vi "DataTranslation_old.vi"() -> (15 "error out":errorcluster={"status"=TRUE, "code"=1172, "source"="Error calling method LvLink2.LvTask.ReadDblData2DAs1D, (System.Reflection.TargetInvocationException: Exception has been thrown by the target of an invocation.\n\tInner Exception: LvLink2.LvException: Timeout) <append><b>LvLink2.LvException</b> in OLReadMultiple2D.vi->DataTranslation_server.vi->Acquire_Data.vi->Get_data.vi->Measurement.vi"})   [LabVIEW 2011]
uses:
  Data_Translation/DataTranslation_global.vi
  Globals/Meas_global.vi
  PWA/PWAtasksGLOBAL.vi
  <userlib>/LV-Link3/PolySubVIs/DtCreateAinChan.vi
  <userlib>/LV-Link3/PolySubVIs/DtOLTimingSetInput.vi
  <userlib>/LV-Link3/PolySubVIs/DtOLReadMultiple2D.vi
  <userlib>/LV-Link3/PolySubVIs/DtOLTriggerDigital.vi
panel:
  in  "error in":errorcluster
  out "AFG error out":errorcluster
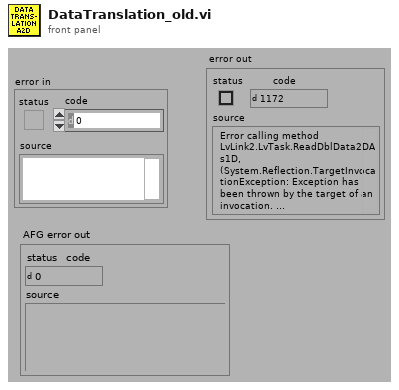
[diagram p1: front panel]
types:
  T1 = typedef "Ch_and_Spans.ctl" = cluster{"high limit (10V)":sgl, "low limit (-10V)":sgl, "Ch No":i16, "Var name":string, "Use Latest Calib":bool}
  T2 = typedef "Trigger_Mode.ctl" = enum16{"Free Running", "Start on Trigger", "Trigger Every Block", "Trigger Every Sample"}
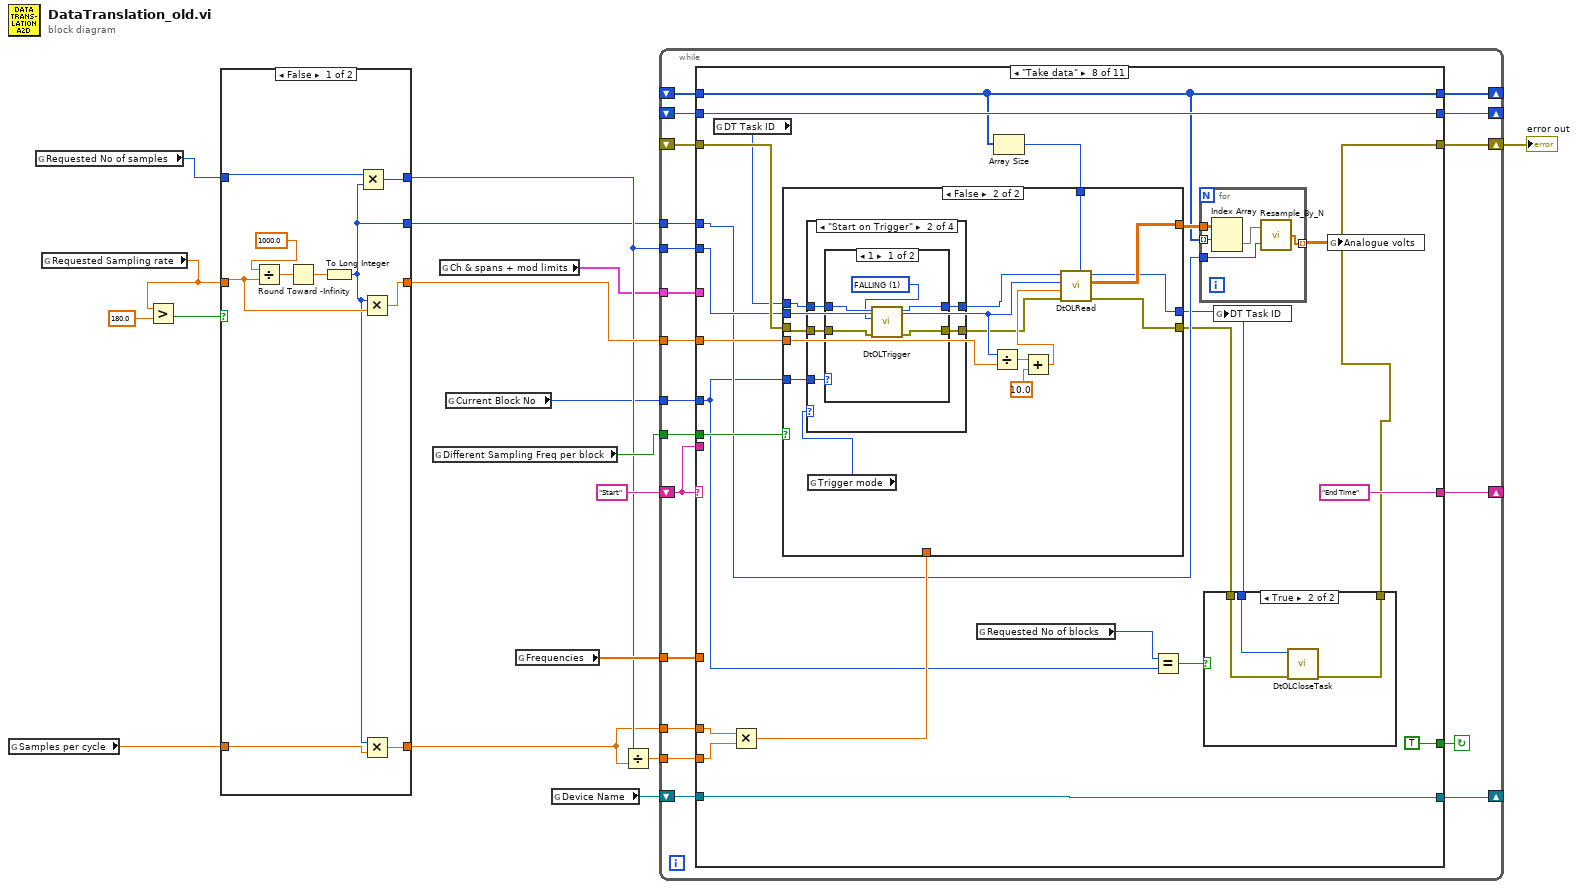
[diagram p0: block diagram]
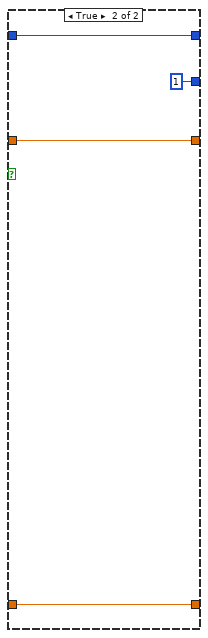
[diagram p2: hidden frame]
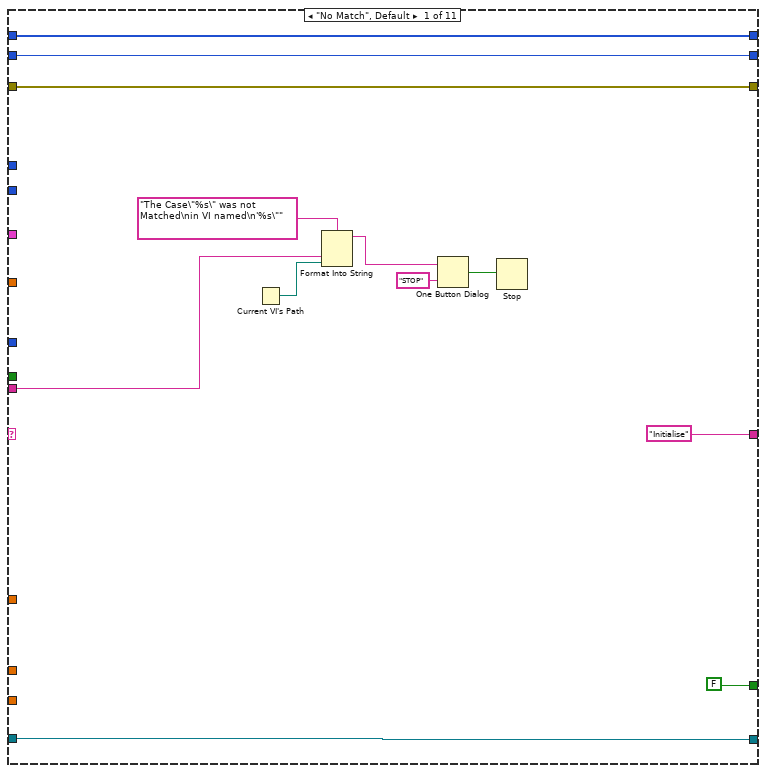
[diagram p3: hidden frame]
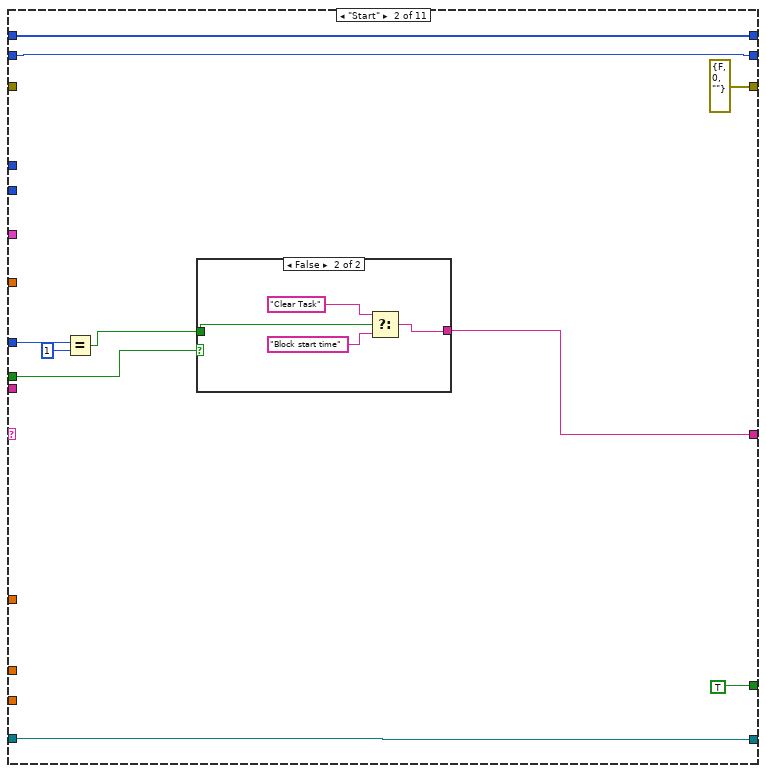
[diagram p4: hidden frame]
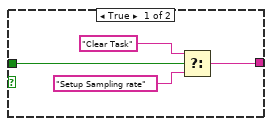
[diagram p5: hidden frame]
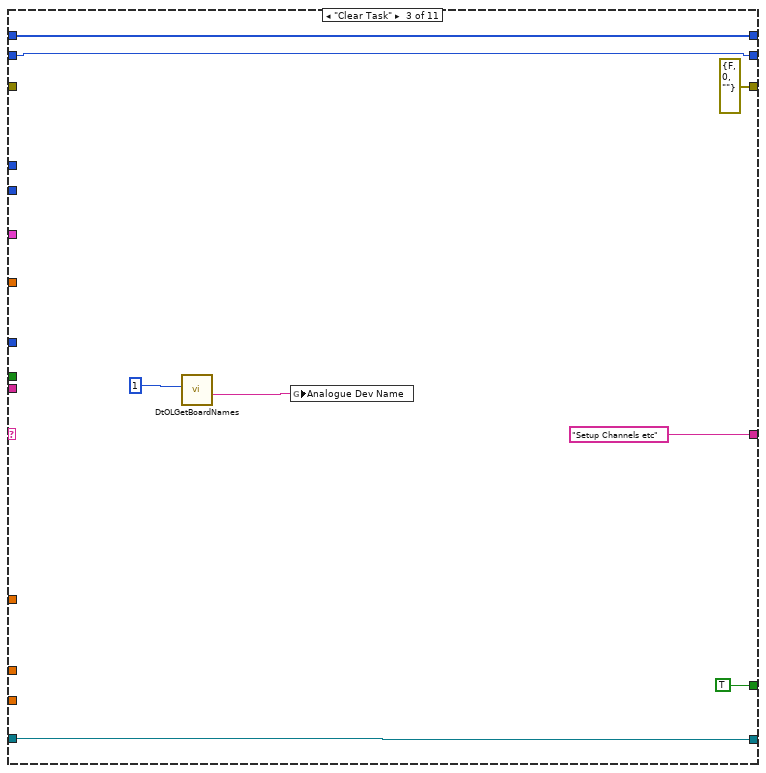
[diagram p6: hidden frame]
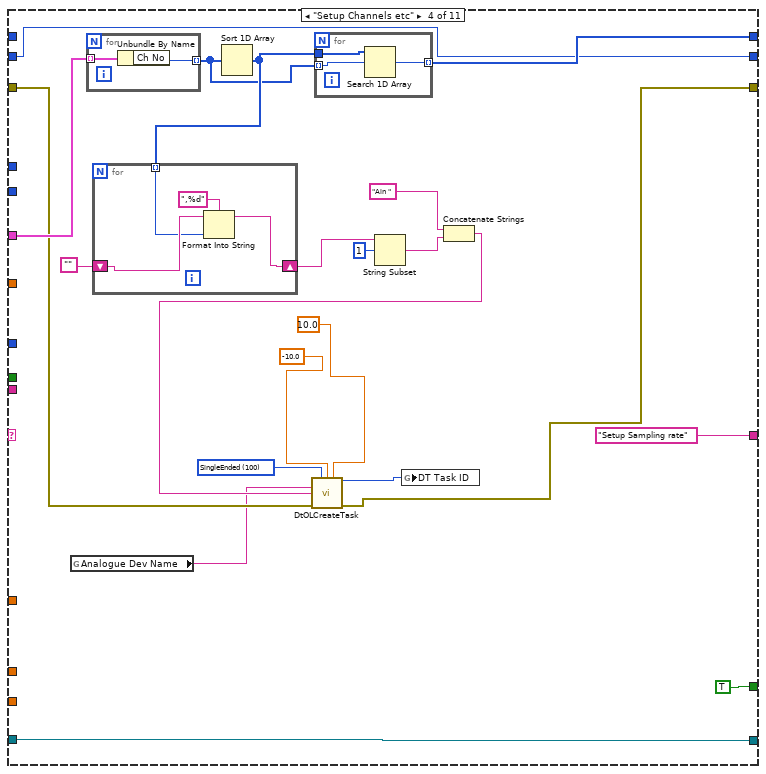
[diagram p7: hidden frame]
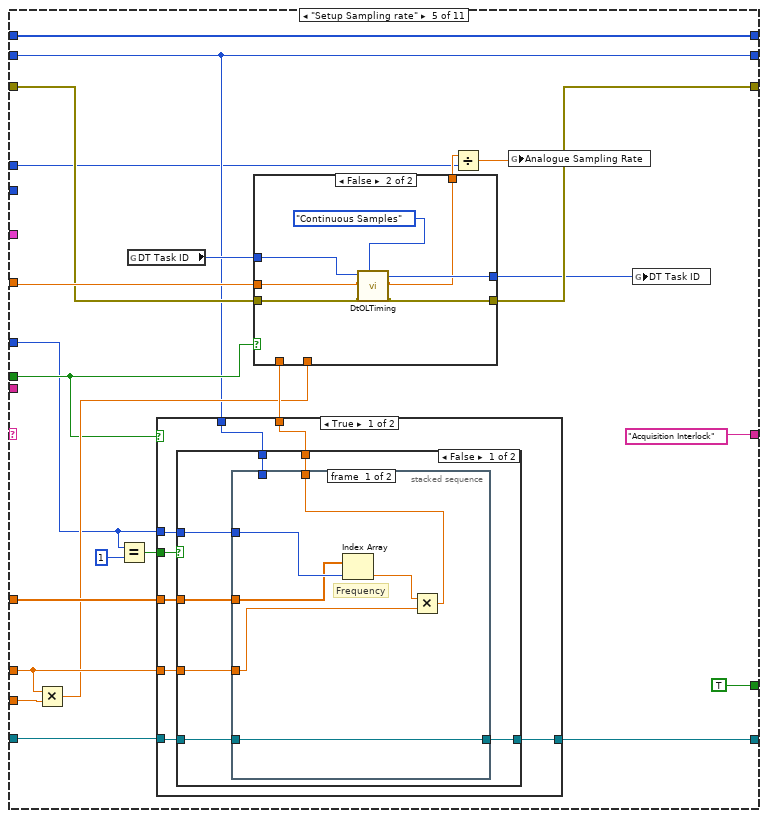
[diagram p8: hidden frame]
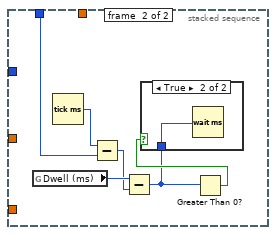
[diagram p9: hidden frame]
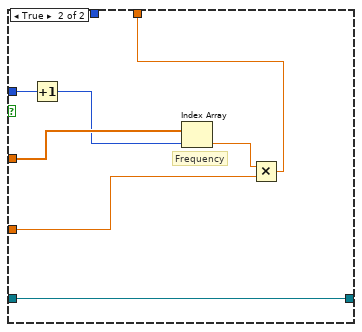
[diagram p11: hidden frame]
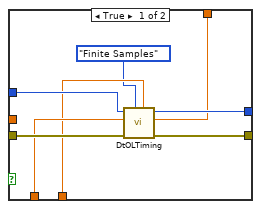
[diagram p13: hidden frame]
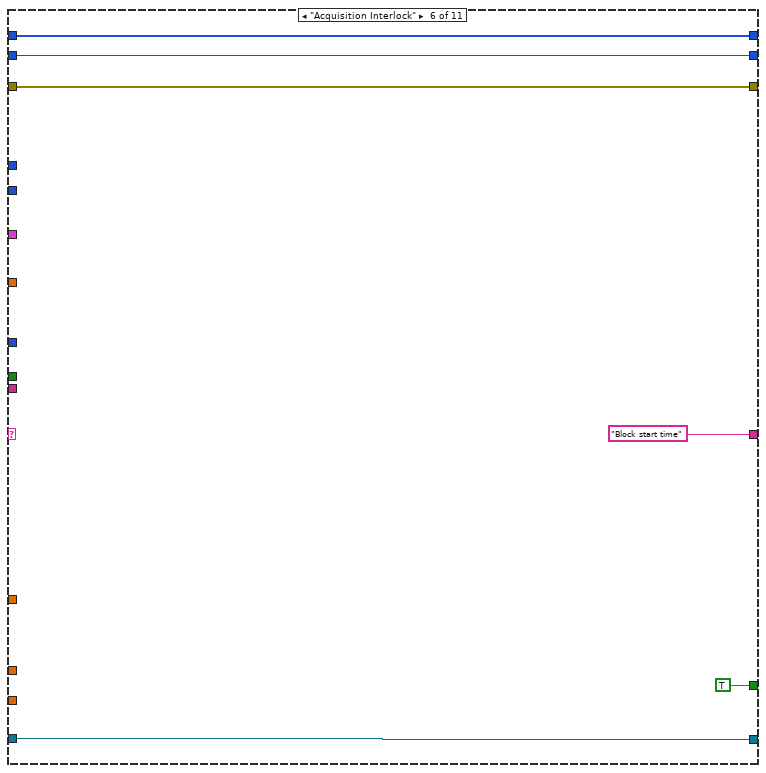
[diagram p14: hidden frame]
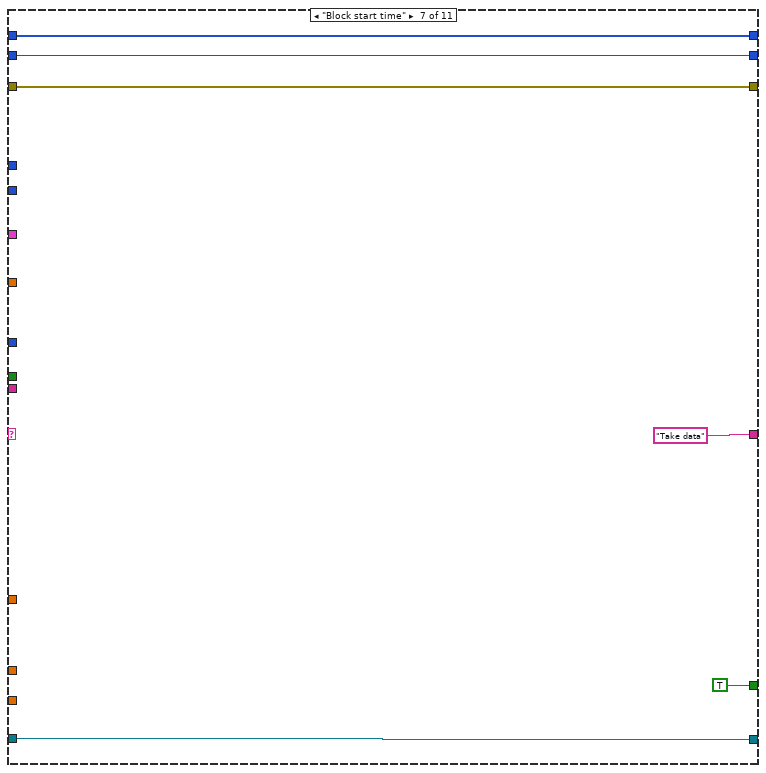
[diagram p15: hidden frame]
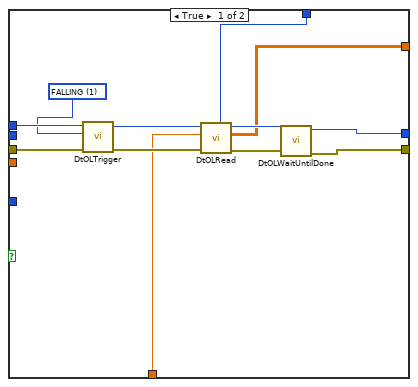
[diagram p17: hidden frame]
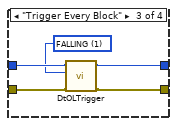
[diagram p20: hidden frame]
diagram:
  n1 = global read "DataTranslation_global.vi" "Samples per cycle"() -> (w6:dbl)
  n2 = global read "Meas_global.vi" "Requested No of samples"() -> (w2:i32)
  n3 = global read "Meas_global.vi" "Requested Sampling rate"() -> (w3:dbl)
  n4 = Greater?(x=w3, y=180.0) -> (0:w10:bool)
  n5 = case shown="False" w10 {
    tunnel: w3 -> [w21 w31]
    tunnel: [w22 w31] -> w9
    tunnel: [w24 w30] -> w8
    tunnel: w2 -> [w23 w30]
    tunnel: [w20 w29] -> w7
    tunnel: w6 -> [w19 w29]
    tunnel: [w18 1] -> w5
    frame False {
      n6 = Divide(x=1000.0, y=w21) -> (x/y=w26:dbl)
      n7 = Round Toward -Infinity(1:w26) -> (0:w25:dbl)
      n8 = To Long Integer(number=w25) -> (32bit integer=w18:i32)
      n9 = Multiply(x=w23, y=w18) -> (x*y=w24:i32)
      n10 = Multiply(x=w18, y=w21) -> (x*y=w22:dbl)
      n11 = Multiply(x=w18, y=w19) -> (x*y=w20:dbl)
    }
    frame True {
    }
  }
  n12 = global read "DataTranslation_global.vi" "Different Sampling Freq per block"() -> (w12:bool)
  n13 = global read "Meas_global.vi" "Ch & spans + mod limits"() -> (w4:T1[])
  n14 = global read "Meas_global.vi" "Current Block No"() -> (w1:i32)
  n15 = global read "DataTranslation_global.vi" "Frequencies"() -> (w13:dbl[])
  n16 = global read "DataTranslation_global.vi" "Device Name"() -> (w14:refnum<visa-resource-name>)
  n17 = Divide(x=w8, y=w7) -> (x/y=w15:dbl)
  n18 = while {
    shift-left: "Start" -> [w49]
    shift-right: [w50] -> _
    shift-right: [w43] -> w16
    shift-left: _ -> [w48]
    tunnel: w9 -> [w47]
    tunnel: w8 -> [w46]
    tunnel: w1 -> [w45]
    tunnel: w4 -> [w44]
    shift-right: [w42] -> _
    shift-left: _ -> [w41]
    tunnel: w7 -> [w39]
    shift-right: [w38] -> _
    shift-left: w14 -> [w40]
    tunnel: w15 -> [w37]
    tunnel: w12 -> [w36]
    tunnel: w13 -> [w35]
    shift-right: [w34] -> _
    shift-left: _ -> [w33]
    tunnel: w5 -> [w32]
    stop <- w51 continue-if-true
    n19 = case shown="\"Take data\"" w49 {
      tunnel: [FALSE TRUE TRUE TRUE TRUE TRUE TRUE TRUE w289 FALSE FALSE] -> w51
      tunnel: ["Initialise" w72 "Setup Channels etc" "Setup Sampling rate" "Acquisition Interlock" "Block start time" "Take data" "End Time" "Add info to block header" ("f") "End" ("f") "End" ("f")] -> w50
      tunnel: w49 -> [w58 _ _ _ _ _ _ _ _ _ _]
      tunnel: [w55 errorcluster {"status"=FALSE, "code"=0, "source"=""} ("error out") errorcluster {"status"=FALSE, "code"=0, "source"=""} ("error out") w92 w141 w199 w206 w209 w291 w304 w335] -> w43
      tunnel: w48 -> [w55 _ _ w93 w139 w199 w206 w227 w291 w304 w335]
      tunnel: w47 -> [_ _ _ _ w140 _ _ w223 _ _ _]
      tunnel: w46 -> [_ _ _ _ _ _ _ w224 _ _ _]
      tunnel: w45 -> [_ w66 _ _ w121 _ _ w207 _ w297 _]
      tunnel: w44 -> [_ _ _ w103 _ _ _ _ _ _ _]
      tunnel: [w54 w70 w87 w100 w136 w197 w203 w216 w290 w303 w334] -> w42
      tunnel: w41 -> [w54 w70 w87 _ w136 w197 w203 w216 w290 w303 w334]
      tunnel: w40 -> [w53 w69 w86 w99 w133 w196 w202 w222 w288 w302 w333]
      tunnel: w35 -> [_ _ _ _ w135 _ _ _ _ w300 _]
      tunnel: w39 -> [_ _ _ _ w129 _ _ w220 _ _ _]
      tunnel: [w53 w69 w86 w99 w132 w196 w202 w222 w288 w301 w333] -> w38
      tunnel: w37 -> [_ _ _ _ w130 _ _ w221 _ _ _]
      tunnel: w36 -> [_ w68 _ _ w127 _ _ w218 w289 _ _]
      tunnel: [w52 w67 w85 w98 w126 w195 w201 w217 w287 w298 w332] -> w34
      tunnel: w33 -> [w52 w67 w85 w98 w126 w195 w201 w217 w287 _ w332]
      tunnel: w32 -> [_ _ _ _ w123 _ _ w214 _ _ _]
      frame "No Match", Default {
        n20 = Current VI's Path() -> (path=w57:path)
        n21 = Format Into String(format string="The Case\"%s\" was not Matched\nin VI named\n'%s\"" ("Format String"), w58, w57) -> (resulting string=w61:string)  [unwired: 2 in, 1 out]
        n22 = One Button Dialog(message=w61, button name ("OK")="STOP") -> (true=w59:bool)
        n23 = Stop(stop? (T)=w59) -> ()
      }
      frame "Start" {
        n24 = Equal?(x=w66, y=1) -> (x = y?=w64:bool)
        n25 = case shown="False" w68 {
          tunnel: w64 -> [w75 w79]
          tunnel: [w74 w78] -> w72
          frame True {
            n26 = Select(t="Clear Task", s=w75, f="Setup Sampling rate") -> (s? t:f=w74:string)
          }
          frame False {
            n27 = Select(t="Clear Task", s=w79, f="Block start time") -> (s? t:f=w78:string)
          }
        }
      }
      frame "Clear Task" {
        n28 = call <userlib>:"DtOLGetBoardNames.vi"("Select Board"=u32 1) -> ("Board Name"=w83:string)  [unwired: 8 in, 2 out]
        n29 = global write "PWAtasksGLOBAL.vi" "Analogue Dev Name"(w83) -> ()
      }
      frame "Setup Channels etc" {
        w94 = 100 items=["SingleEnded"=100, "Differential"=101] ("Channel Type")
        n30 = global read "PWAtasksGLOBAL.vi" "Analogue Dev Name"() -> (w90:string)
        n31 = for {
          tunnel: w103 -> [w115] mode=indexing
          tunnel: [w114] -> w101 mode=indexing
          n32 = Unbundle By Name(w115) -> ("Ch No"=w114:i16)
        }
        n33 = Sort 1D Array(array=w101) -> (sorted array=w102:i16[])
        n34 = for {
          shift-right: [w117] -> w108
          shift-left: "" -> [w118]
          tunnel: w102 -> [w116] mode=indexing
          n35 = Format Into String(format string=",%d", initial string=w118, w116) -> (resulting string=w117:string)  [unwired: 1 in, 1 out]
        }
        n36 = for {
          tunnel: w102 -> [w113]
          tunnel: w101 -> [w112] mode=indexing
          tunnel: [w111] -> w100 mode=indexing
          n37 = Search 1D Array(1D array=w113, element=w112) -> (index of element=w111:i32)  [unwired: 1 in]
        }
        n38 = String Subset(string=w108, offset (0)=1) -> (substring=w105:string)  [unwired: 1 in]
        n39 = Concatenate Strings("Ain ", w105) -> (w97:string)
        n40 = call-poly <userlib>:"DtOLCreateTask.vi"("Channel Type"=w94, "Range Min"=-10.0, "Range Max"=10.0, "Board Name"=w90, "Channel"=w97, "error in (no error)"=w93) -> ("Task out"=w91:i32, "error out"=w92:errorcluster)  [unwired: 7 in, 1 out]
        n41 = global write "DataTranslation_global.vi" "DT Task ID"(w91) -> ()
      }
      frame "Setup Sampling rate" {
        n42 = Multiply(x=w129, y=w130) -> (x*y=w128:dbl)
        n43 = Equal?(x=w121, y=1) -> (x = y?=w125:bool)
        n44 = global read "DataTranslation_global.vi" "DT Task ID"() -> (w137:i32)
        n45 = case shown="True" w127 {
          tunnel: w135 -> [w146 _]
          tunnel: [w150 w178] -> w134
          tunnel: w129 -> [w149 w178]
          tunnel: w121 -> [w148 _]
          tunnel: w133 -> [w147 w179]
          tunnel: [w145 w179] -> w132
          tunnel: w126 -> [w144 _]
          tunnel: w125 -> [w143 _]
          frame True {
            n46 = case shown="False" w143 {
              tunnel: [w157 w174] -> w150
              tunnel: w149 -> [w156 w173]
              tunnel: w148 -> [w151 w175]
              tunnel: w147 -> [w155 w172]
              tunnel: w146 -> [w154 w176]
              tunnel: [w153 w172] -> w145
              tunnel: w144 -> [w152 _]
              frame False {
                n47 = stacked-sequence {
                  tunnel: [w163 _] -> w157
                  tunnel: w156 -> [w162 _]
                  tunnel: w151 -> [w161 _]
                  tunnel: w155 -> [w158 _]
                  tunnel: w154 -> [w160 _]
                  tunnel: [w158 _] -> w153
                  tunnel: w152 -> [_ w168]
                  frame #0 {
                    # "Frequency"
                    n48 = Index Array(array=w160, index=w161) -> (element=w159:dbl)
                    n49 = Multiply(x=w159, y=w162) -> (x*y=w163:dbl)
                  }
                  frame #1 {
                    n50 = global read "DataTranslation_global.vi" "Dwell (ms)"() -> (w167:u32)
                    n51 = Tick Count (ms)() -> (millisecond timer value=w169:u32)
                    n52 = Subtract(x=w169, y=w168) -> (x-y=w166:u32)
                    n53 = Subtract(x=w167, y=w166) -> (x-y=w164:u32)
                    n54 = Greater Than 0?(x=w164) -> (x > 0?=w165:bool)
                    n55 = case shown="True" w165 {
                      tunnel: w164 -> [_ w170]
                      frame False {
                      }
                      frame True {
                        n56 = Wait (ms)(milliseconds to wait=w170) -> ()  [unwired: 1 out]
                      }
                    }
                  }
                }
              }
              frame True {
                # "Frequency"
                n57 = Increment(x=w175) -> (x+1=w171:i32)
                n58 = Index Array(array=w176, index=w171) -> (element=w177:dbl)
                n59 = Multiply(x=w177, y=w173) -> (x*y=w174:dbl)
              }
            }
          }
          frame False {
          }
        }
        n60 = case shown="False" w127 {
          tunnel: [w184 w189] -> w141
          tunnel: w140 -> [_ w192]
          tunnel: [w183 w191] -> w124
          tunnel: w139 -> [w185 w190]
          tunnel: [w186 w194] -> w138
          tunnel: w137 -> [w187 w193]
          tunnel: w134 -> [w182 _]
          tunnel: w128 -> [w181 _]
          frame True {
            n61 = call-poly <userlib>:"DtOLTiming.vi"("Samples Per Channel"=w181, "Sample Mode"=enum16{"Finite Samples", "Continuous Samples"}."Finite Samples", "error in (no error)"=w185, "Sample Freq (Hz)"=w182, "Task in"=w187) -> ("error out"=w184:errorcluster, "Actual Sample Freq"=w183:dbl, "Task out"=w186:i32)  [unwired: 3 in, 1 out]
          }
          frame False {
            n62 = call-poly <userlib>:"DtOLTiming.vi"("Sample Mode"=enum16{"Finite Samples", "Continuous Samples"}."Continuous Samples", "error in (no error)"=w190, "Sample Freq (Hz)"=w192, "Task in"=w193) -> ("error out"=w189:errorcluster, "Actual Sample Freq"=w191:dbl, "Task out"=w194:i32)  [unwired: 4 in, 1 out]
          }
        }
        n63 = Divide(x=w124, y=w123) -> (x/y=w122:dbl)
        n64 = global write "Meas_global.vi" "Analogue Sampling Rate"(w122) -> ()
        n65 = global write "DataTranslation_global.vi" "DT Task ID"(w138) -> ()
      }
      frame "Acquisition Interlock" {
      }
      frame "Block start time" {
      }
      frame "Take data" {
        n66 = global read "DataTranslation_global.vi" "DT Task ID"() -> (w226:i32)
        n67 = Multiply(x=w220, y=w221) -> (x*y=w219:dbl)
        n68 = global read "Meas_global.vi" "Requested No of blocks"() -> (w213:i32)
        n69 = Array Size(array=w216) -> (size(s)=w215:i32)
        n70 = case shown="False" w218 {
          tunnel: w227 -> [w245 w255]
          tunnel: [w242 w249] -> w210
          tunnel: [w239 w247] -> w212
          tunnel: w226 -> [w238 w256]
          tunnel: [w236 w248] -> w225
          tunnel: w224 -> [_ w252]
          tunnel: w223 -> [_ w260]
          tunnel: w219 -> [w235 _]
          tunnel: w207 -> [_ w254]
          tunnel: w215 -> [w234 w246]
          frame True {
            w237 = 1 items=["RISING", "FALLING"] ("External Trigger Polarity")
            n71 = call-poly <userlib>:"DtOLTrigger.vi"("error in (no error)"=w245, "External Trigger Polarity"=w237, "Task in"=w238) -> ("error out"=w244:errorcluster, "Task out"=w241:i32)  [unwired: 7 in]
            n72 = call-poly <userlib>:"DtOLRead.vi"("Number Chan to Read"=w234, "error in (no error)"=w244, "Samples Per Channel"=w235, "Task in"=w241) -> ("error out"=w243:errorcluster, "2D Data out"=w236:dbl[][], "Task out"=w240:i32)  [unwired: 3 in, 2 out]
            n73 = call <userlib>:"DtOLWaitUntilDone.vi"("error in"=w243, "Task in"=w240) -> ("error out"=w242:errorcluster, "Task out"=w239:i32)  [unwired: 8 in]
          }
          frame False {
            n74 = global read "Meas_global.vi" "Trigger mode"() -> (w257:T2)
            n75 = case shown="\"Start on Trigger\"" w257 {
              tunnel: [w262 w264 w278 w281] -> w253
              tunnel: w256 -> [w262 w266 w279 w281]
              tunnel: [w261 w263 w275 w280] -> w250
              tunnel: w255 -> [w261 w265 w276 w280]
              tunnel: w254 -> [_ w267 _ _]
              frame "Free Running" {
              }
              frame "Start on Trigger" {
                n76 = case shown="1" w267 {
                  tunnel: w266 -> [w272 w274]
                  tunnel: w265 -> [w270 w273]
                  tunnel: [w268 w274] -> w264
                  tunnel: [w269 w273] -> w263
                  frame 1 {
                    w271 = 1 items=["RISING", "FALLING"] ("External Trigger Polarity")
                    n77 = call-poly <userlib>:"DtOLTrigger.vi"("error in (no error)"=w270, "External Trigger Polarity"=w271, "Task in"=w272) -> ("error out"=w269:errorcluster, "Task out"=w268:i32)  [unwired: 7 in]
                  }
                  frame 2, Default {
                  }
                }
              }
              frame "Trigger Every Block" {
                w277 = 1 items=["RISING", "FALLING"] ("External Trigger Polarity")
                n78 = call-poly <userlib>:"DtOLTrigger.vi"("error in (no error)"=w276, "External Trigger Polarity"=w277, "Task in"=w279) -> ("error out"=w275:errorcluster, "Task out"=w278:i32)  [unwired: 7 in]
              }
              frame "Trigger Every Sample" {
              }
            }
            n79 = Divide(x=w252, y=w260) -> (x/y=w258:dbl)
            n80 = Add(x=w258, y=10.0) -> (x+y=w251:dbl)
            n81 = call-poly <userlib>:"DtOLRead.vi"("Number Chan to Read"=w246, "error in (no error)"=w250, "Timeout"=w251, "Samples Per Channel"=w252, "Task in"=w253) -> ("error out"=w249:errorcluster, "2D Data out"=w248:dbl[][], "Task out"=w247:i32)  [unwired: 2 in, 2 out]
          }
        }
        n82 = Equal?(x=w213, y=w207) -> (x = y?=w211:bool)
        n83 = for {
          tunnel: w216 -> [w286] mode=indexing
          tunnel: w225 -> [w285]
          tunnel: [w283] -> w208 mode=indexing
          tunnel: w214 -> [w282]
          n84 = Index Array(array=w285, index (row)=w286) -> (element=w284:dbl[])  [unwired: 1 in]
          n85 = call "Resample_By_N.vi"("Resample Factor"=w282, "Array In"=w284) -> ("Array Out"=w283:dbl[])
        }
        n86 = case shown="True" w211 {
          tunnel: w212 -> [_ w233]
          tunnel: w210 -> [w230 w232]
          tunnel: [w230 w231] -> w209
          frame False {
          }
          frame True {
            n87 = call <userlib>:"DtOLCloseTask.vi"("Error in"=w232, "Task in"=w233) -> ("Error Out"=w231:errorcluster)  [unwired: 9 in]
          }
        }
        n88 = global write "DataTranslation_global.vi" "DT Task ID"(w212) -> ()
        n89 = global write "Meas_global.vi" "Analogue volts"(w208) -> ()
      }
      frame "End Time" {
        # "Final transpose to get 2D data output correctly"
      }
      frame "Add info to block header" {
        n90 = global read "Meas_global.vi" "Requested No of blocks"() -> (w293:i32)
        n91 = global read "DataTranslation_global.vi" "Amplitudes"() -> (w294:dbl[])
        n92 = Index Array(array=w294, index=w297) -> ()  [unwired: 1 out]
        n93 = Index Array(array=w300, index=w297) -> ()  [unwired: 1 out]
        n94 = Equal?(x=w297, y=w293) -> (x = y?=w299:bool)
        n95 = case shown="False" w299 {
          tunnel: w302 -> [w319 w329]
          tunnel: [w310 w327] -> w301
          tunnel: [w312 w328] -> w295
          tunnel: w300 -> [w315 w330]
          tunnel: w294 -> [w316 w331]
          tunnel: w297 -> [w314 _]
          tunnel: [w316 w331] -> _
          tunnel: [w315 w330] -> _
          tunnel: "error in" -> [w307 w325]
          frame False {
            w320 = "SOUR1" ("input 1")
            w323 = ":%s:FREQ %.;%g;"  # Frequency Command
            w324 = ":%s:VOLT %.;%g;"  # Amplitude Command
            n96 = Increment(x=w314) -> (x+1=w313:i32)
            n97 = Index Array(array=w316, index=w313) -> (element=w318:dbl)
            n98 = Index Array(array=w315, index=w313) -> (element=w317:dbl)
            n99 = Format Into String(format string=w323, w320, w317) -> (resulting string=w321:string)  [unwired: 2 in, 1 out]
            n100 = Format Into String(format string=w324, initial string=w321, w320, w318) -> (resulting string=w322:string)  [unwired: 1 in, 1 out]
            n101 = VISA Write(VISA resource name=w319, write buffer=w322, error in (no error)=w307) -> (VISA resource name out=w311:refnum<visa-resource-name>, error out=w309:errorcluster)  [unwired: 1 out]
            n102 = VISA Write(VISA resource name=w311, write buffer="OUTP1:STAT ON", error in (no error)=w309) -> (VISA resource name out=w310:refnum<visa-resource-name>, error out=w312:errorcluster)  [unwired: 1 out]
          }
          frame True {
            n103 = VISA Write(VISA resource name=w329, write buffer="OUTP1:STAT OFF", error in (no error)=w325) -> (VISA resource name out=w327:refnum<visa-resource-name>, error out=w328:errorcluster)  [unwired: 1 out]
          }
        }
        "AFG error out" <- w295
        n104 = Tick Count (ms)() -> (millisecond timer value=w298:u32)
      }
      frame "Extra case" {
      }
    }
  }
  "error out" <- w16
